vi "test2.vi"(5 "Action":T1, 8 "error in (no error)":errorcluster, 9 "Cluster In":T2, 11 "reference in":refnum<k24>) -> (0 "error out":errorcluster, 1 "Cluster out":T2, 3 "reference out":refnum<k24>)   [LabVIEW 2018]
uses:
  Thorlabs Translation Stages/Controls/Translation Stage Cluster.ctl
  General/Controls/Translation Stage Types.ctl
  Thorlabs Translation Stages/Controls/Motion Translation Module Control.ctl
  C:/Project/SerialSectionOCT/SerialSectOCT/Labview Software/Thorlabs.MotionControl.Controls.dll
  Thorlabs.MotionControl.Controls.dll
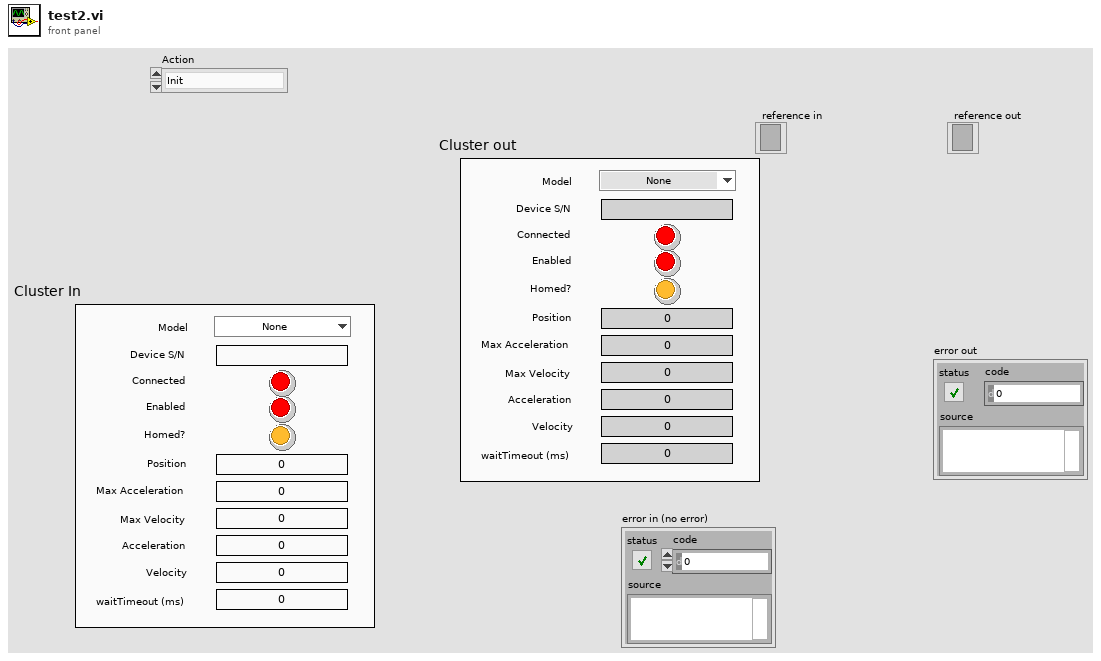
[diagram p1: front panel]
types:
  T1 = typedef "Motion Translation Module Control.ctl" = enum16{"Init", "Home", "Status", "Velocity/Accel", "Position", "Jog", "Stop", "Uninit", "Enable", "Disable"}
  T2 = typedef "Translation Stage Cluster.ctl" = cluster{"Position":dbl, "Is.Enabled?":bool, "Is.Connected?":bool, "Device SN":string, "AccelerationMaximum":dbl, "VelocityMaximum":dbl, "Acceleration":dbl, "Velocity":dbl, "waitTimeout (ms)":i32, "Model":T3, "Is.Homed?":bool}
  T3 = typedef "Translation Stage Types.ctl" = enum16{"None", "Thorlabs LTS", "Thorlabs MLJ"}
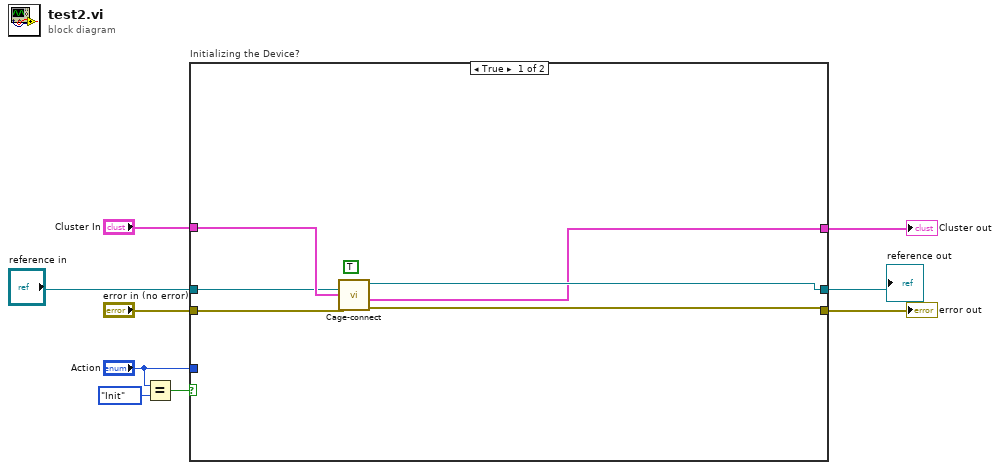
[diagram p0: block diagram]
diagram:
  n1 = Equal?(x="Action", y=Motion_Translation_Module_Control."Init") -> (x = y?=w2:bool)
  n2 = case "Initializing the Device?" shown="True" w2 {
    tunnel: "reference in" -> [w13 w17]
    tunnel: [w11 w17] -> w9
    tunnel: [w10 w16] -> w8
    tunnel: [w12 w18] -> w7
    tunnel: "error in (no error)" -> [w15 w18]
    tunnel: "Cluster In" -> [w14 w16]
    tunnel: "Action" -> [_ _]
    frame True {
      (unwired) TRUE ("Enable?")
      n3 = call "Cage-connect.vi"("error in (no error)"=w15, "Cluster in"=w14, "reference in"=w13) -> ("error out"=w12:errorcluster, "Cluster out"=w10:T2, "reference out"=w11:refnum<k24>)  [unwired: 5 in, 1 out]
    }
    frame False {
    }
  }
  "Cluster out" <- w8
  "error out" <- w7
  "reference out" <- w9
